vi "PutString.vi"(8 "error in (no error)":errorcluster, 10 "string":string, 11 "MsgPackSerializer in":refnum<class "MsgPackSerializer.lvclass">) -> (0 "error out":errorcluster, 3 "MsgPackSerializer out":refnum<class "MsgPackSerializer.lvclass">)   [LabVIEW 2015, in "MsgPackSerializer.lvclass"]
uses:
  MsgPackSerializer.lvclass
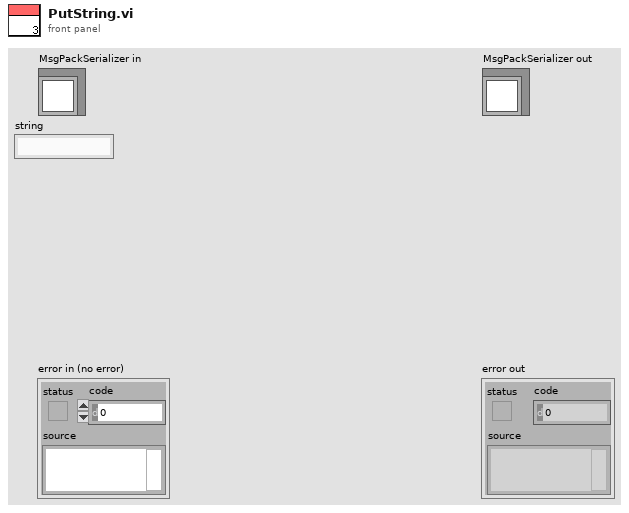
[diagram p1: front panel]
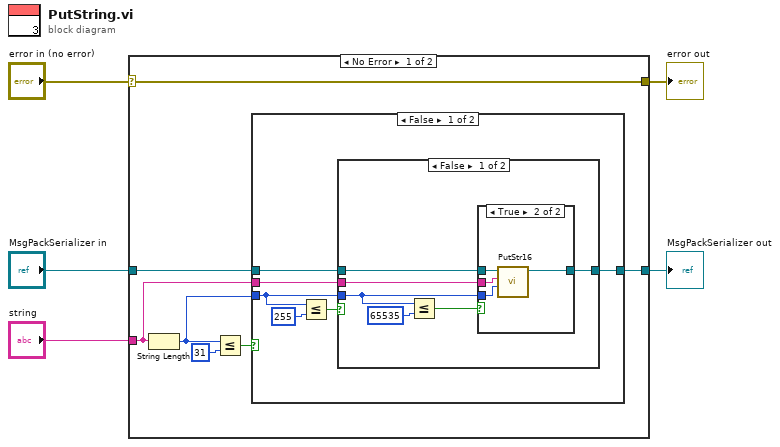
[diagram p0: block diagram]
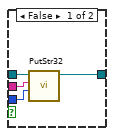
[diagram p2: hidden frame]
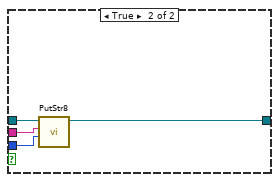
[diagram p3: hidden frame]
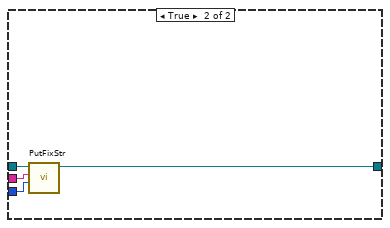
[diagram p4: hidden frame]
diagram:
  n1 = case shown="No Error" "error in (no error)" {
    selector: "error in (no error)" -> [w12 w42]
    tunnel: [w12 w42] -> w4
    tunnel: [w7 w41] -> w2
    tunnel: "MsgPackSerializer in" -> [w8 w41]
    tunnel: "string" -> [w6 _]
    frame No Error {
      n2 = String Length(string=w6) -> (length=w11:i32)
      n3 = Less Or Equal?(x=w11, y=31) -> (x <= y?=w10:bool)
      n4 = case shown="False" w10 {
        tunnel: w8 -> [w15 w40]
        tunnel: w6 -> [w16 w39]
        tunnel: w11 -> [w14 w38]
        tunnel: [w13 w37] -> w7
        frame False {
          n5 = Less Or Equal?(x=w14, y=255) -> (x <= y?=w17:bool)
          n6 = case shown="False" w17 {
            tunnel: w16 -> [w22 w36]
            tunnel: w15 -> [w21 w35]
            tunnel: w14 -> [w20 w33]
            tunnel: [w19 w34] -> w13
            frame False {
              n7 = Less Or Equal?(x=w20, y=65535) -> (x <= y?=w23:bool)
              n8 = case shown="True" w23 {
                tunnel: w22 -> [w27 w32]
                tunnel: w21 -> [w26 w31]
                tunnel: w20 -> [w28 w30]
                tunnel: [w25 w29] -> w19
                frame False {
                  n9 = call "PutStr32.vi"("Size"=w28, "string"=w27, "MsgPackSerializer in"=w26) -> ("MsgPackSerializer out"=w25:refnum<class "MsgPackSerializer.lvclass">)  [unwired: 7 in, 1 out]
                }
                frame True {
                  n10 = call "PutStr16.vi"("Size"=w30, "string"=w32, "MsgPackSerializer in"=w31) -> ("MsgPackSerializer out"=w29:refnum<class "MsgPackSerializer.lvclass">)  [unwired: 7 in, 1 out]
                }
              }
            }
            frame True {
              n11 = call "PutStr8.vi"("Size"=w33, "string"=w36, "MsgPackSerializer in"=w35) -> ("MsgPackSerializer out"=w34:refnum<class "MsgPackSerializer.lvclass">)  [unwired: 7 in, 1 out]
            }
          }
        }
        frame True {
          n12 = call "PutFixStr.vi"("Size"=w38, "string"=w39, "MsgPackSerializer in"=w40) -> ("MsgPackSerializer out"=w37:refnum<class "MsgPackSerializer.lvclass">)  [unwired: 7 in, 1 out]
        }
      }
    }
    frame Error {
    }
  }
  "error out" <- w4
  "MsgPackSerializer out" <- w2
